vi "GRIMMMeasurementGFV.vi"(8 "error in (no error)":errorcluster, 10 "Variant in":variant, 11 "GRIMMMeasEnum":T2=enum."InsertMeasurement") -> (0 "error out":errorcluster, 3 "Variant out":variant)   [LabVIEW 2013]
doc: "Use this template to build a VI to use as a subVI."
uses:
  GRIMMmeasurementEnum.ctl
  GRIMMErrorMessage.ctl
  GRIMMmeasurementCluster.ctl
  GRIMMCurrentCountsPerBin.ctl
  GRIMMstatusEnum.ctl
panel:
  out "data":T1 items=["New SELF-TEST: Fault Self-Test"=128, "No Memory Card"=64, "Check Nozzle: Whirls > 5%"=32, "No Operation: Battery Capacity = 0%"=16, "Please Recharge: Battery Capacity < 10%"=8, "Pump Current too High - Motor Current Imot > 100%"=4, "Flow-Error: Volume flow control out of control range"=3, "Check Filter Imot < 20% "=2, "Check Filter Imot > 60%"=1, "No Error :)"=0]
  out "element 4":dbl
  out "element 3":dbl
  out "element 2":dbl
  out "element":dbl
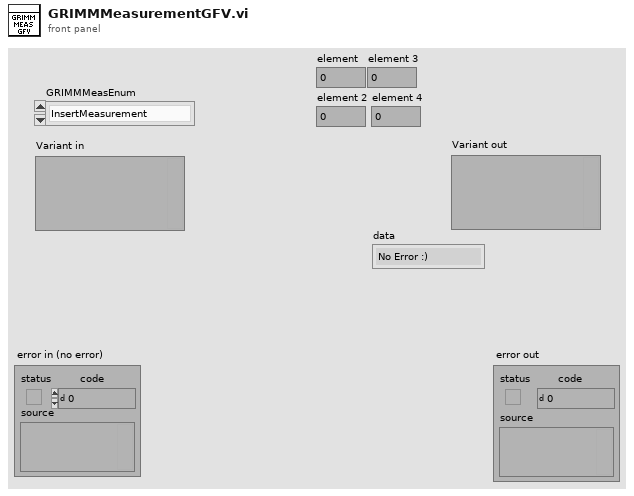
[diagram p1: front panel]
types:
  T1 = typedef "GRIMMErrorMessage.ctl" = u16
  T2 = typedef "GRIMMmeasurementEnum.ctl" = enum16{"Get CurrentNvsBin WebService", "Save Raw to file", "Get NvsDiameter", "Get DNDlogDPVsDiameter", "Get CountsVsTime", "Get Raw Data", "InsertMeasurement", "Init"}
  T3 = typedef "GRIMMmeasurementCluster.ctl" = cluster{"Threshold Bin size":dbl[], "Measurement Data":i32[]}
  T4 = typedef "GRIMMstatusEnum.ctl" = enum16{"Get Pump Current", "Get Power Supply Type", "Get Battery Power", "Get Error message", "Get Instrument DateTime", "Insert Status Data", "Init"}
  T5 = enum16{"open", "replace", "create", "open or create", "replace or create", "replace or create with confirmation"}
  T6 = typedef "GRIMMCurrentCountsPerBin.ctl" = cluster{"dateTime":string, "CountsPerBin":dbl[]}
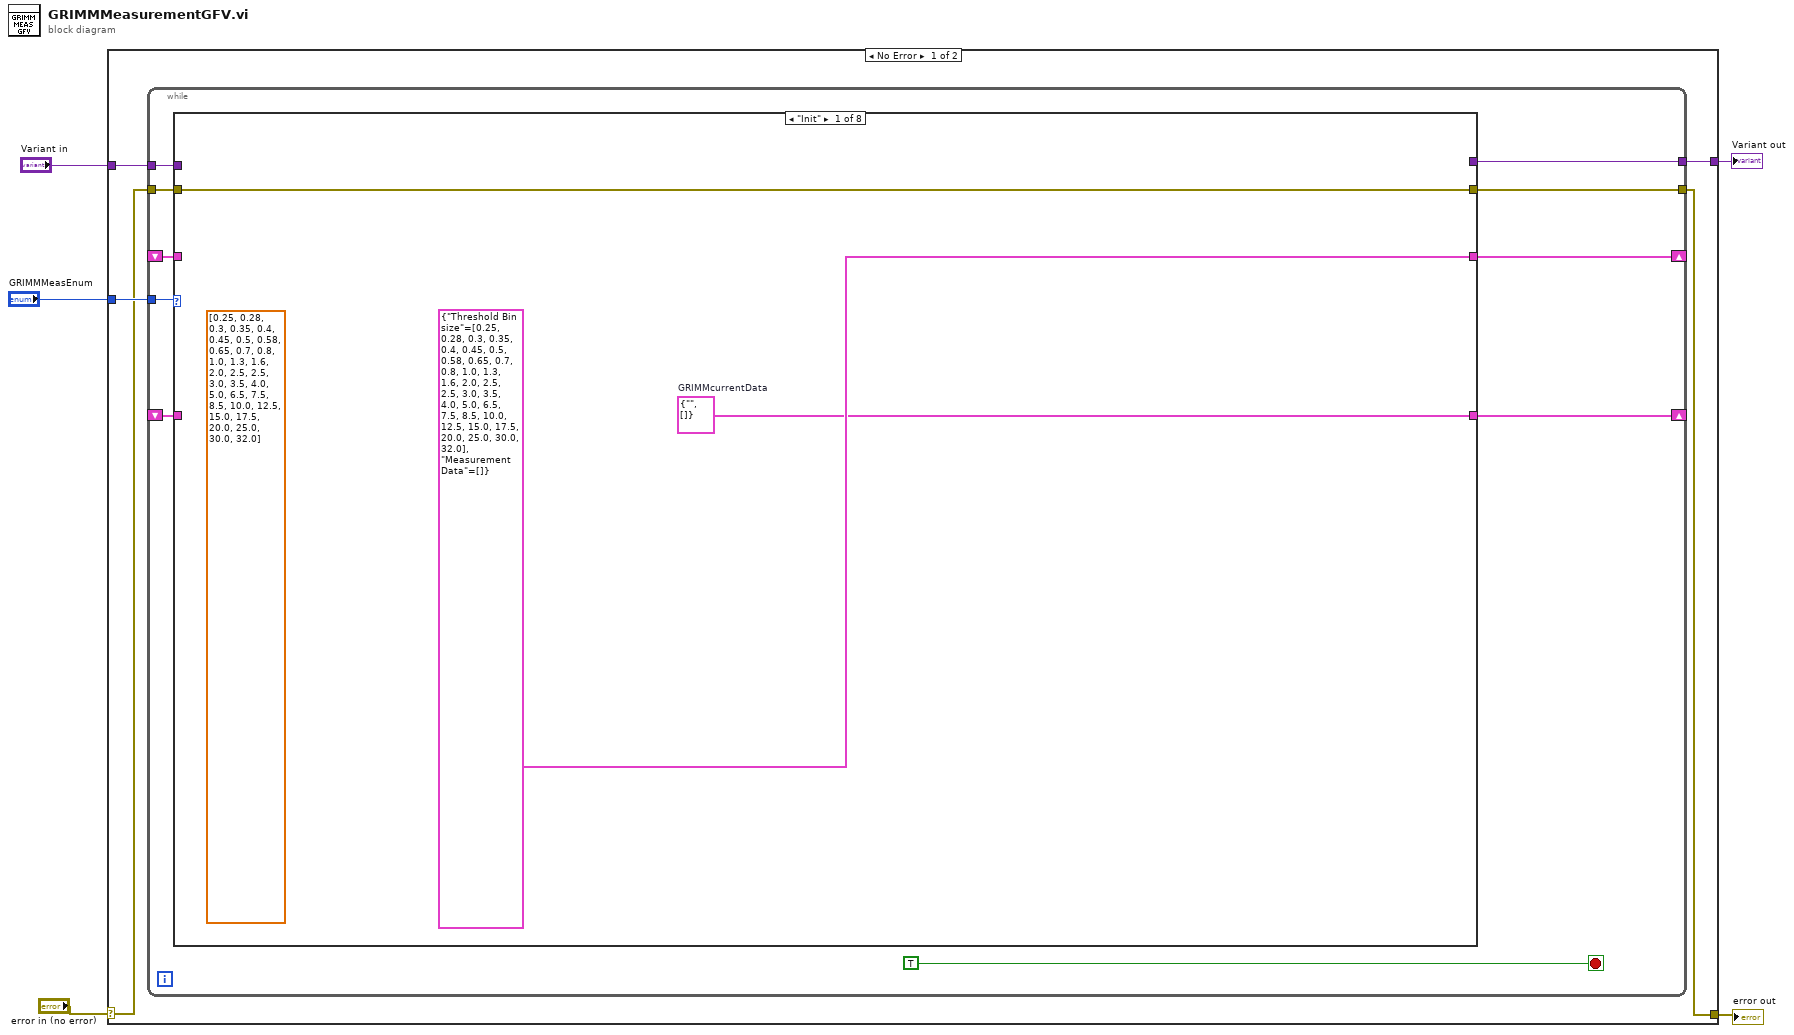
[diagram p0: block diagram]
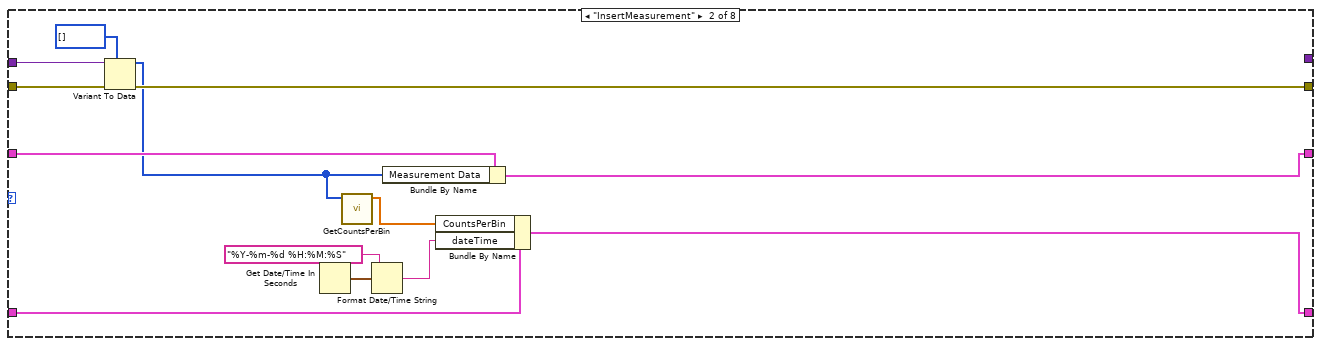
[diagram p2: hidden frame]
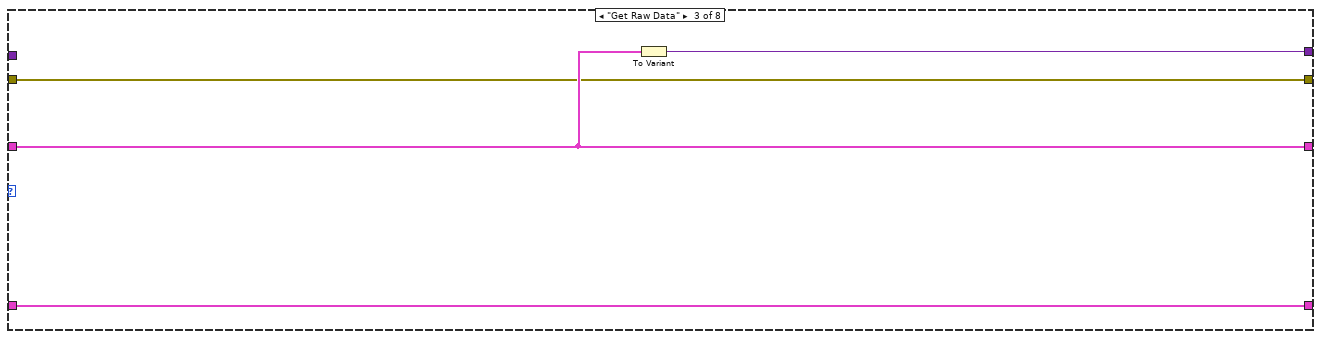
[diagram p3: hidden frame]
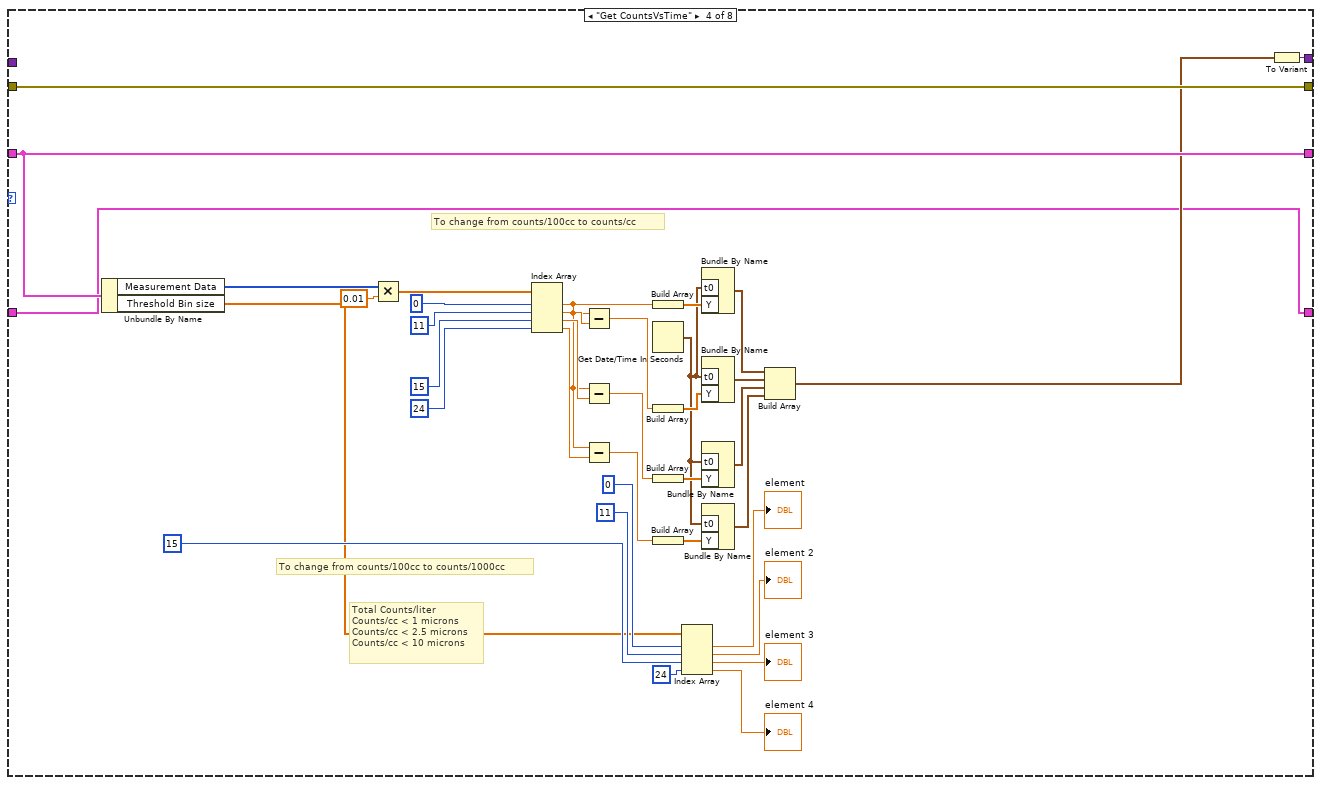
[diagram p4: hidden frame]
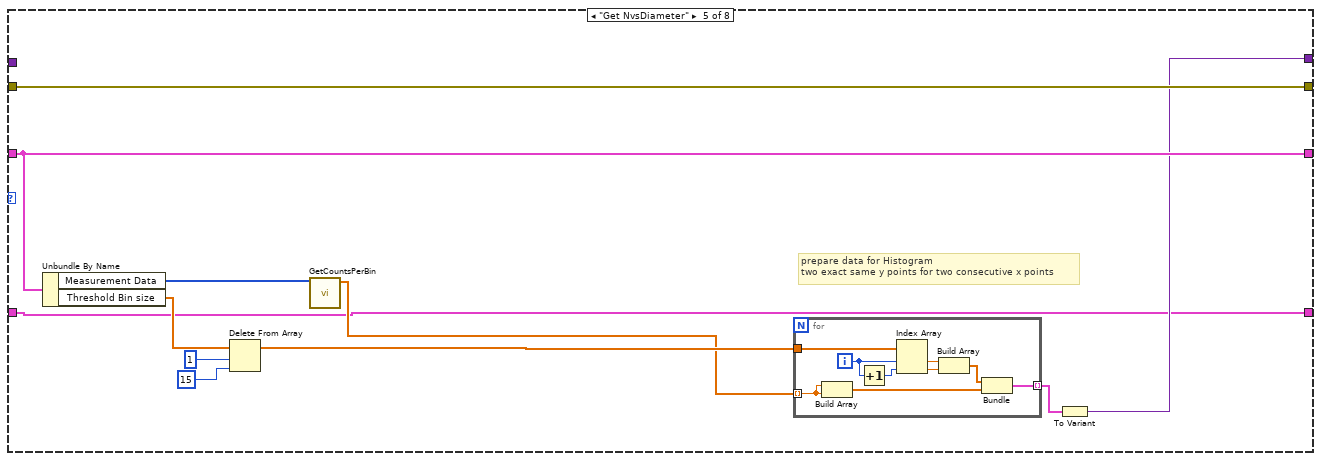
[diagram p5: hidden frame]
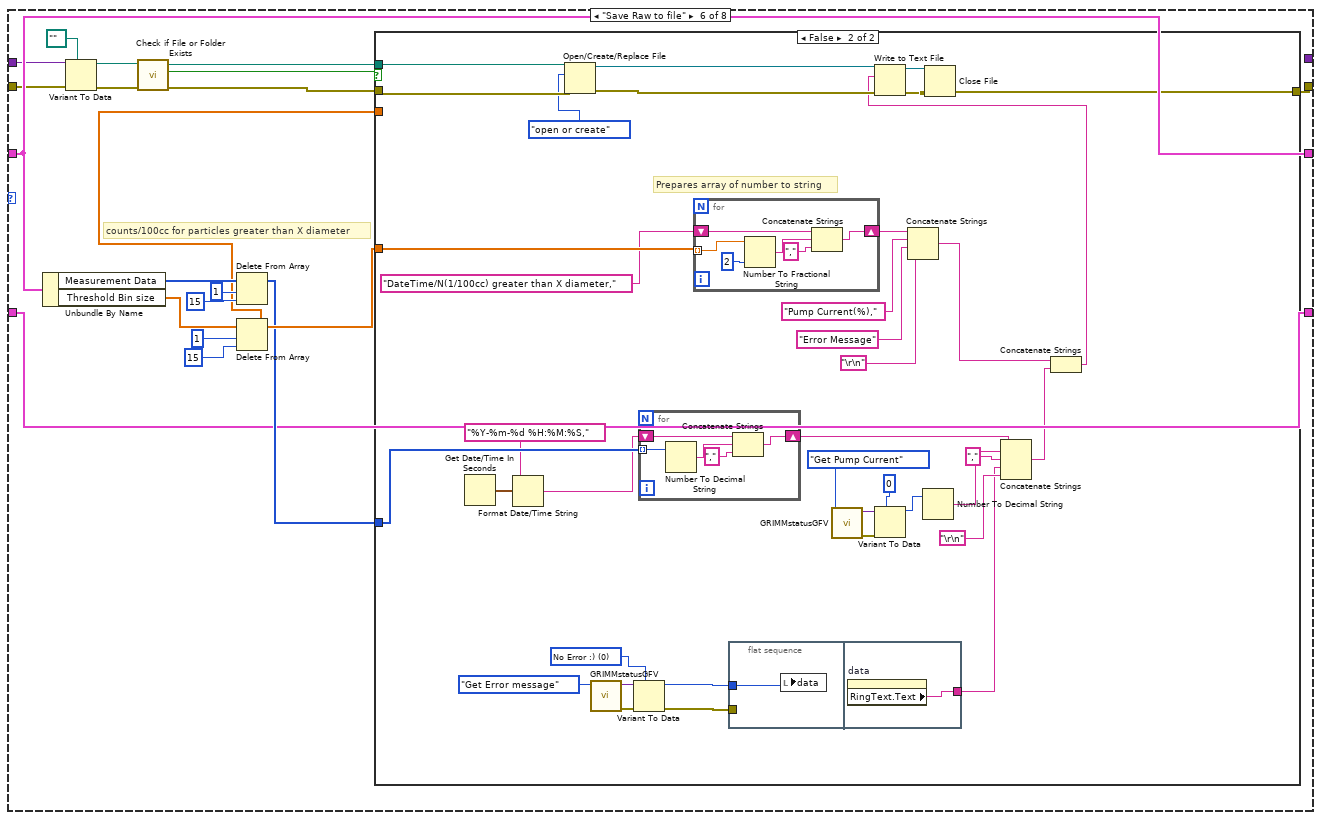
[diagram p6: hidden frame]
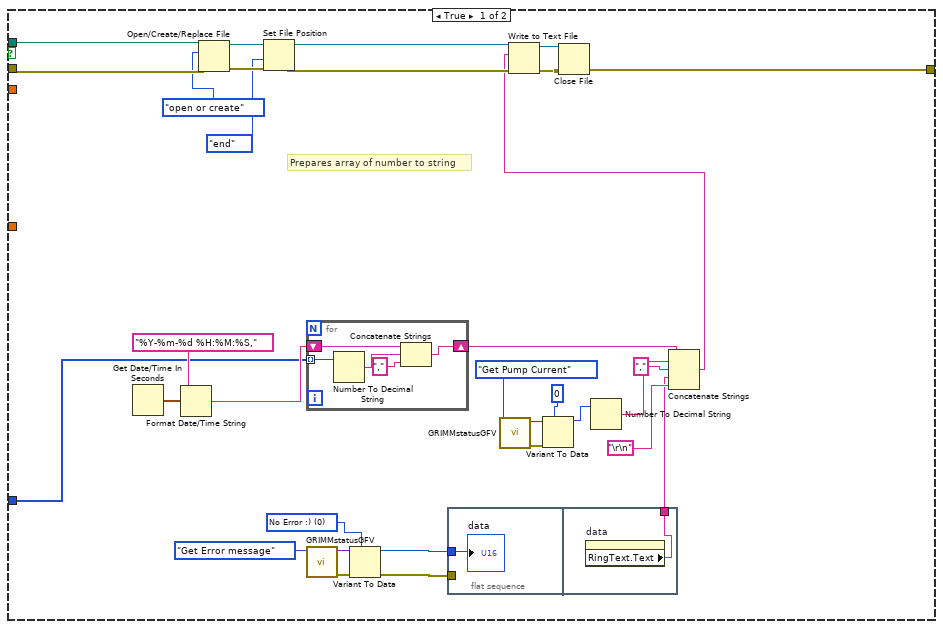
[diagram p7: hidden frame]
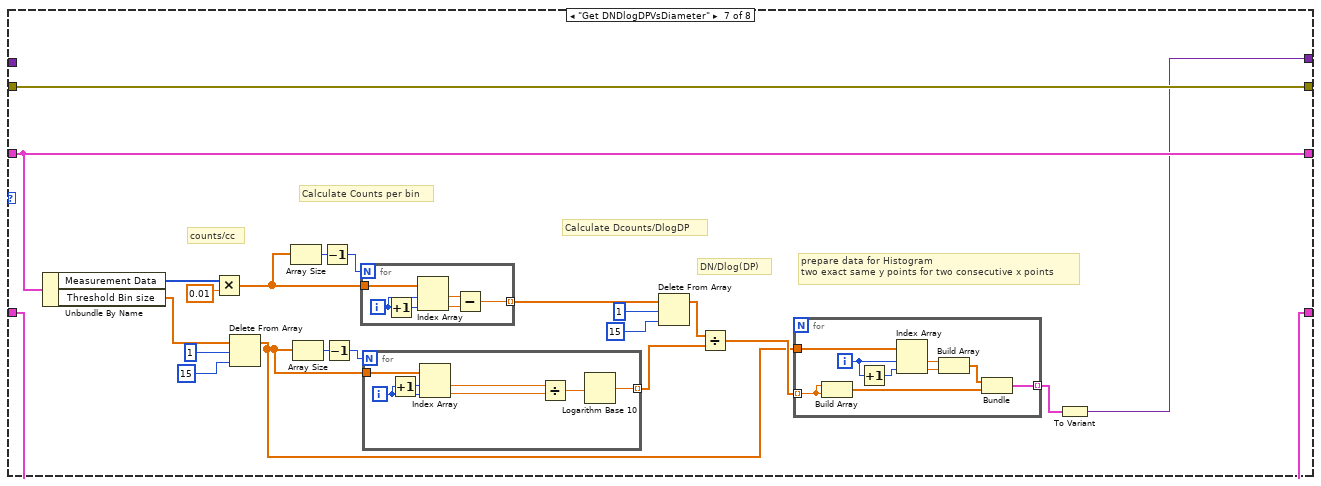
[diagram p8: hidden frame]
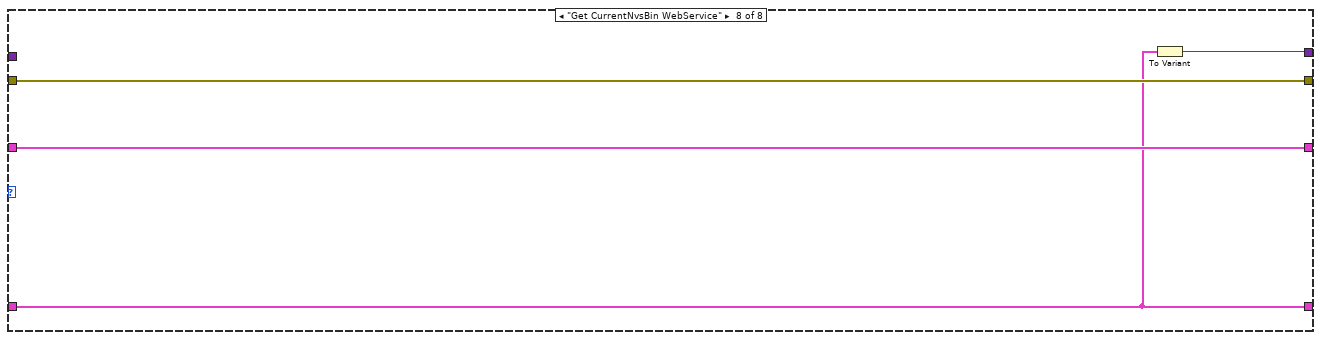
[diagram p9: hidden frame]
diagram:
  n1 = case shown="No Error" "error in (no error)" {
    selector: "error in (no error)" -> [w8 w255]
    tunnel: [w7 w255] -> w4
    tunnel: "GRIMMMeasEnum" -> [w10 _]
    tunnel: "Variant in" -> [w9 w254]
    tunnel: [w6 w254] -> w1
    frame No Error {
      n2 = while {
        tunnel: w10 -> [w19]
        shift-right: [w18] -> _
        shift-left: _ -> [w17]
        tunnel: w9 -> [w16]
        tunnel: w8 -> [w15]
        tunnel: [w14] -> w7
        tunnel: [w13] -> w6
        shift-right: [w12] -> _
        shift-left: _ -> [w11]
        stop <- TRUE stop-if-true
        n3 = case shown="\"Init\"" w19 {
          tunnel: [T3 {"Threshold Bin size"=[0.25, 0.28, 0.3, 0.35, 0.4, 0.45, 0.5, 0.58, 0.65, 0.7, 0.8, 1.0, 1.3, 1.6, 2.0, 2.5, 2.5, 3.0, 3.5, 4.0, 5.0, 6.5, 7.5, 8.5, 10.0, 12.5, 15.0, 17.5, 20.0, 25.0, 30.0, 32.0], "Measurement Data"=[]} w35 w40 w75 w87 w116 w226 w253] -> w18
          tunnel: w17 -> [_ w36 w40 w75 w87 w116 w226 w253]
          tunnel: w16 -> [_ w33 _ _ _ w108 _ _]
          tunnel: w15 -> [w23 w34 w38 w76 w88 w109 w227 w252]
          tunnel: [w23 w31 w38 w76 w88 w101 w227 w252] -> w14
          tunnel: [_ _ w39 w77 w81 _ w207 w251] -> w13
          tunnel: [w21 w24 w37 w41 w78 w98 w206 w250] -> w12
          tunnel: w11 -> [_ w27 w37 w41 w78 w98 w206 w250]
          frame "Init" {
            w21 = T6 {"dateTime"="", "CountsPerBin"=[]}  # GRIMMcurrentData
            (unwired) dbl[] [0.25, 0.28, 0.3, 0.35, 0.4, 0.45, 0.5, 0.58, 0.65, 0.7, 0.8, 1.0, 1.3, 1.6, 2.0, 2.5, 2.5, 3.0, 3.5, 4.0, 5.0, 6.5, 7.5, 8.5, 10.0, 12.5, 15.0, 17.5, 20.0, 25.0, 30.0, 32.0] ("Threshold Bin size")
          }
          frame "InsertMeasurement" {
            n4 = Variant To Data(error in=w34, type=i32[] [] ("f"), Variant=w33) -> (data=w30:i32[], error out=w31:errorcluster)
            n5 = Get Date/Time In Seconds() -> (seconds since 1Jan1904=w29:timestamp)
            n6 = call "GetCountsPerBin.vi"("Counts until bin number"=w30) -> ("Counts per Bin"=w26:dbl[])  [unwired: 10 in]
            n7 = Format Date/Time String(time format string (%c)="%Y-%m-%d %H:%M:%S", seconds (now)=w29) -> (date/time string=w25:string)  [unwired: 1 in]
            n8 = Bundle By Name(cluster=w36, "Measurement Data"=w30) -> (w35:T3)
            n9 = Bundle By Name(cluster=w27, "CountsPerBin"=w26, "dateTime"=w25) -> (w24:T6)
          }
          frame "Get Raw Data" {
            n10 = To Variant(anything=w40) -> (Variant=w39:variant)
          }
          frame "Get CountsVsTime" {
            # "To change from counts/100cc to counts/1000cc"
            # "To change from counts/100cc to counts/cc"
            # "Total Counts/liter\nCounts/cc < 1 microns\nCounts/cc < 2.5 microns\nCounts/cc < 10 microns"
            n11 = Unbundle By Name(w75) -> ("Measurement Data"=w74:i32[], "Threshold Bin size"=w63:dbl[])
            n12 = Multiply(x=w74, y=0.01) -> (x*y=w72:dbl[])
            n13 = Index Array(array=w72, index #1=0 ("index"), index #2=11 ("index"), index #3=15 ("index"), index #4=24 ("index")) -> (element #1=w55:dbl, element #2=w58:dbl, element #3=w57:dbl, element #4=w56:dbl)
            n14 = Subtract(x=w55, y=w58) -> (x-y=w48:dbl)
            n15 = Subtract(x=w55, y=w57) -> (x-y=w47:dbl)
            n16 = Subtract(x=w55, y=w56) -> (x-y=w46:dbl)
            n17 = Build Array(w55) -> (w54:dbl[])
            n18 = Get Date/Time In Seconds() -> (seconds since 1Jan1904=w42:timestamp)
            n19 = Build Array(w48) -> (w51:dbl[])
            n20 = Build Array(w47) -> (w50:dbl[])
            n21 = Build Array(w46) -> (w49:dbl[])
            n22 = Index Array(array=w63, index #1=0 ("index"), index #2=11 ("index"), index #3=15 ("index"), index #4=24 ("index")) -> (element #1=→"element":dbl, element #2=→"element 2":dbl, element #3=→"element 3":dbl, element #4=→"element 4":dbl)
            n23 = Bundle By Name("t0"=w42, "Y"=w54) -> (w52:waveform(dbl))  [unwired: 1 in]
            n24 = Bundle By Name("t0"=w42, "Y"=w51) -> (w45:waveform(dbl))  [unwired: 1 in]
            n25 = Bundle By Name("t0"=w42, "Y"=w50) -> (w44:waveform(dbl))  [unwired: 1 in]
            n26 = Bundle By Name("t0"=w42, "Y"=w49) -> (w43:waveform(dbl))  [unwired: 1 in]
            n27 = Build Array(w52, w45, w44, w43) -> (w53:waveform(dbl)[])
            n28 = To Variant(anything=w53) -> (Variant=w77:variant)
          }
          frame "Get NvsDiameter" {
            # "prepare data for Histogram\ntwo exact same y points for two consecutive x points"
            n29 = Unbundle By Name(w87) -> ("Measurement Data"=w80:i32[], "Threshold Bin size"=w84:dbl[])
            n30 = Delete From Array(array=w84, length=1, index=15) -> (array with subset deleted=w83:dbl[])  [unwired: 1 out]
            n31 = call "GetCountsPerBin.vi"("Counts until bin number"=w80) -> ("Counts per Bin"=w79:dbl[])  [unwired: 10 in]
            n32 = for {
              tunnel: w79 -> [w94] mode=indexing
              tunnel: w83 -> [w97]
              tunnel: [w89] -> w82 mode=indexing
              i -> [w96]
              n33 = Build Array(w94, w94) -> (w90:dbl[])
              n34 = Increment(x=w96) -> (x+1=w95:i32)
              n35 = Index Array(array=w97, index #1=w96, index #2=w95) -> (element #1=w93:dbl, element #2=w92:dbl)
              n36 = Build Array(w93, w92) -> (w91:dbl[])
              n37 = Bundle(w91, w90) -> (w89:cluster{dbl[], dbl[]})  [unwired: 1 in]
            }
            n38 = To Variant(anything=w82) -> (Variant=w81:variant)
          }
          frame "Save Raw to file" {
            # "counts/100cc for particles greater than X diameter"
            n39 = Unbundle By Name(w116) -> ("Measurement Data"=w110:i32[], "Threshold Bin size"=w111:dbl[])
            n40 = Variant To Data(error in=w109, type=path "" ("GRIMM File Path"), Variant=w108) -> (data=w105:path, error out=w106:errorcluster)
            n41 = call <vilib>:"Check if File or Folder Exists.vi"("error in (no error)"=w106, "path"=w105) -> ("error out"=w103:errorcluster, "file or folder exists?"=w104:bool, "dup path"=w102:path)  [unwired: 7 in]
            n42 = Delete From Array(array=w110, length=1, index=15) -> (array with subset deleted=w99:i32[])  [unwired: 1 out]
            n43 = Delete From Array(array=w111, length=1, index=15) -> (array with subset deleted=w100:dbl[])  [unwired: 1 out]
            n44 = case shown="False" w104 {
              tunnel: w103 -> [w148 w192]
              tunnel: w102 -> [w147 w191]
              tunnel: [w146 w190] -> w101
              tunnel: w100 -> [_ _]
              tunnel: w100 -> [_ w186]
              tunnel: w99 -> [w121 w183]
              frame True {
                w126 = T1 0 items=["New SELF-TEST: Fault Self-Test"=128, "No Memory Card"=64, "Check Nozzle: Whirls > 5%"=32, "No Operation: Battery Capacity = 0%"=16, "Please Recharge: Battery Capacity < 10%"=8, "Pump Current too High - Motor Current Imot > 100%"=4, "Flow-Error: Volume flow control out of control range"=3, "Check Filter Imot < 20% "=2, "Check Filter Imot > 60%"=1, "No Error :)"=0] ("Error Messages")
                # "Prepares array of number to string"
                n45 = Get Date/Time In Seconds() -> (seconds since 1Jan1904=w137:timestamp)
                n46 = Format Date/Time String(time format string (%c)="%Y-%m-%d %H:%M:%S,", seconds (now)=w137) -> (date/time string=w135:string)  [unwired: 1 in]
                n47 = Open/Create/Replace File(file path (use dialog)=w147, error in=w148, operation (0:open)=T5."open or create") -> (refnum out=w143:refnum<file>, error out=w144:errorcluster)  [unwired: 3 in, 1 out]
                n48 = Set File Position(refnum=w143, from (0:start)=enum16{"start", "end", "current"}."end", error in=w144) -> (refnum out=w138:refnum<file>, error out=w139:errorcluster)  [unwired: 1 in]
                n49 = for {
                  tunnel: w121 -> [w155] mode=indexing
                  shift-right: [w151] -> w130
                  shift-left: w135 -> [w153]
                  n50 = Number To Decimal String(number=w155) -> (decimal integer string=w152:string)  [unwired: 1 in]
                  n51 = Concatenate Strings(w153, w152, "," ("string")) -> (w151:string)
                }
                n52 = call "GRIMMstatusGFV.vi"("GrimmStatusEnum"=GRIMMstatusEnum."Get Error message") -> ("error out"=w125:errorcluster, "Variant out"=w127:variant)  [unwired: 9 in]
                n53 = Variant To Data(error in=w125, type=w126, Variant=w127) -> (data=w118:T1, error out=w119:errorcluster)
                n54 = flat-sequence {
                  tunnel: w119 -> [_]
                  tunnel: w118 -> [w149]
                  tunnel: [w150] -> w117
                  frame #0 {
                    "data" <- w149
                  }
                  frame #1 {
                    n55 = property on="data" class="Ring (strict)"() -> ("RingText.Text"=w150:string)  [unwired: 2 in, 2 out]
                  }
                }
                n56 = call "GRIMMstatusGFV.vi"("GrimmStatusEnum"=GRIMMstatusEnum."Get Pump Current") -> ("error out"=w132:errorcluster, "Variant out"=w133:variant)  [unwired: 9 in]
                n57 = Variant To Data(error in=w132, type=0 ("Pump Current %"), Variant=w133) -> (data=w129:i32)  [unwired: 1 out]
                n58 = Number To Decimal String(number=w129) -> (decimal integer string=w128:string)  [unwired: 1 in]
                n59 = Concatenate Strings(w130, w128, "," ("string"), w117, "\r\n") -> (w120:string)
                n60 = Write to Text File(file (use dialog)=w138, text=w120, error in=w139) -> (refnum out=w140:refnum<file>, error out=w141:errorcluster)  [unwired: 1 in, 1 out]
                n61 = Close File(refnum=w140, error in=w141) -> (error out=w146:errorcluster)  [unwired: 1 out]
              }
              frame False {
                w161 = T1 0 items=["New SELF-TEST: Fault Self-Test"=128, "No Memory Card"=64, "Check Nozzle: Whirls > 5%"=32, "No Operation: Battery Capacity = 0%"=16, "Please Recharge: Battery Capacity < 10%"=8, "Pump Current too High - Motor Current Imot > 100%"=4, "Flow-Error: Volume flow control out of control range"=3, "Check Filter Imot < 20% "=2, "Check Filter Imot > 60%"=1, "No Error :)"=0] ("Error Messages")
                # "Prepares array of number to string"
                n62 = Get Date/Time In Seconds() -> (seconds since 1Jan1904=w180:timestamp)
                n63 = Format Date/Time String(time format string (%c)="%Y-%m-%d %H:%M:%S,", seconds (now)=w180) -> (date/time string=w178:string)  [unwired: 1 in]
                n64 = Open/Create/Replace File(file path (use dialog)=w191, error in=w192, operation (0:open)=T5."open or create") -> (refnum out=w185:refnum<file>, error out=w184:errorcluster)  [unwired: 3 in, 1 out]
                n65 = call "GRIMMstatusGFV.vi"("GrimmStatusEnum"=GRIMMstatusEnum."Get Error message") -> ("error out"=w160:errorcluster, "Variant out"=w162:variant)  [unwired: 9 in]
                n66 = Variant To Data(error in=w160, type=w161, Variant=w162) -> (data=w157:T1, error out=w158:errorcluster)
                n67 = for {
                  tunnel: w183 -> [w199] mode=indexing
                  shift-right: [w195] -> w172
                  shift-left: w178 -> [w197]
                  n68 = Number To Decimal String(number=w199) -> (decimal integer string=w196:string)  [unwired: 1 in]
                  n69 = Concatenate Strings(w197, w196, "," ("string")) -> (w195:string)
                }
                n70 = for {
                  tunnel: w186 -> [w205] mode=indexing
                  shift-right: [w200] -> w182
                  shift-left: "DateTime/N(1/100cc) greater than X diameter," -> [w202]
                  n71 = Number To Fractional String(number=w205, precision (6)=i16 2) -> (F-format string=w201:string)  [unwired: 2 in]
                  n72 = Concatenate Strings(w202, w201, "," ("string")) -> (w200:string)
                }
                n73 = flat-sequence {
                  tunnel: w158 -> [_]
                  tunnel: w157 -> [w193]
                  tunnel: [w194] -> w156
                  frame #0 {
                    n74 = local write "data"(w193) -> ()
                  }
                  frame #1 {
                    n75 = property on="data" class="Ring (strict)"() -> ("RingText.Text"=w194:string)  [unwired: 2 in, 2 out]
                  }
                }
                n76 = call "GRIMMstatusGFV.vi"("GrimmStatusEnum"=GRIMMstatusEnum."Get Pump Current") -> ("error out"=w175:errorcluster, "Variant out"=w176:variant)  [unwired: 9 in]
                n77 = Variant To Data(error in=w175, type=0 ("Pump Current %"), Variant=w176) -> (data=w171:i32)  [unwired: 1 out]
                n78 = Concatenate Strings(w182, "Pump Current(%)," ("string"), "Error Message" ("string"), "\r\n") -> (w165:string)
                n79 = Number To Decimal String(number=w171) -> (decimal integer string=w170:string)  [unwired: 1 in]
                n80 = Concatenate Strings(w172, w170, "," ("string"), w156, "\r\n") -> (w164:string)
                n81 = Concatenate Strings(w165, w164) -> (w163:string)
                n82 = Write to Text File(file (use dialog)=w185, text=w163, error in=w184) -> (refnum out=w187:refnum<file>, error out=w188:errorcluster)  [unwired: 1 in, 1 out]
                n83 = Close File(refnum=w187, error in=w188) -> (error out=w190:errorcluster)  [unwired: 1 out]
              }
            }
          }
          frame "Get DNDlogDPVsDiameter" {
            # "counts/cc"
            # "DN/Dlog(DP)"
            # "Calculate Dcounts/DlogDP"
            # "prepare data for Histogram\ntwo exact same y points for two consecutive x points"
            # "Calculate Counts per bin"
            n84 = Unbundle By Name(w226) -> ("Measurement Data"=w214:i32[], "Threshold Bin size"=w218:dbl[])
            n85 = Multiply(x=w214, y=0.01) -> (x*y=w213:dbl[])
            n86 = Delete From Array(array=w218, length=1, index=15) -> (array with subset deleted=w209:dbl[])  [unwired: 1 out]
            n87 = Array Size(array=w213) -> (size(s)=w225:i32)
            n88 = Array Size(array=w209) -> (size(s)=w216:i32)
            n89 = Decrement(x=w225) -> (x-1=w224:i32)
            n90 = Decrement(x=w216) -> (x-1=w217:i32)
            n91 = for {
              N: w224 -> [_]
              tunnel: w213 -> [w249]
              tunnel: [w244] -> w223 mode=indexing
              i -> [w248]
              n92 = Increment(x=w248) -> (x+1=w247:i32)
              n93 = Index Array(array=w249, index #1=w248, index #2=w247) -> (element #1=w245:dbl, element #2=w246:dbl)
              n94 = Subtract(x=w245, y=w246) -> (x-y=w244:dbl)
            }
            n95 = for {
              N: w217 -> [_]
              tunnel: w209 -> [w243]
              tunnel: [w237] -> w211 mode=indexing
              i -> [w242]
              n96 = Increment(x=w242) -> (x+1=w241:i32)
              n97 = Index Array(array=w243, index #1=w241, index #2=w242) -> (element #1=w240:dbl, element #2=w239:dbl)
              n98 = Divide(x=w240, y=w239) -> (x/y=w238:dbl)
              n99 = Logarithm Base 10(1:w238) -> (0:w237:dbl)
            }
            n100 = Delete From Array(array=w223, length=1, index=15) -> (array with subset deleted=w212:dbl[])  [unwired: 1 out]
            n101 = Divide(x=w212, y=w211) -> (x/y=w210:dbl[])
            n102 = for {
              tunnel: w210 -> [w233] mode=indexing
              tunnel: w209 -> [w236]
              tunnel: [w228] -> w208 mode=indexing
              i -> [w235]
              n103 = Build Array(w233, w233) -> (w229:dbl[])
              n104 = Increment(x=w235) -> (x+1=w234:i32)
              n105 = Index Array(array=w236, index #1=w235, index #2=w234) -> (element #1=w232:dbl, element #2=w231:dbl)
              n106 = Build Array(w232, w231) -> (w230:dbl[])
              n107 = Bundle(w230, w229) -> (w228:cluster{dbl[], dbl[]})  [unwired: 1 in]
            }
            n108 = To Variant(anything=w208) -> (Variant=w207:variant)
          }
          frame "Get CurrentNvsBin WebService" {
            n109 = To Variant(anything=w250) -> (Variant=w251:variant)
          }
        }
      }
    }
    frame Error {
    }
  }
  "error out" <- w4
  "Variant out" <- w1
